vi "Extrae_Wait.vi"(10 "String":string="Wait for Temperature, Field, Timeout 300sec, Continue") -> (1 "Array":string[](array[string]))   [LabVIEW 2017]
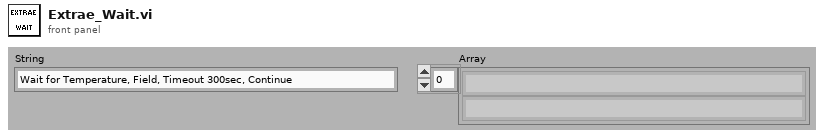
[diagram p1: front panel]
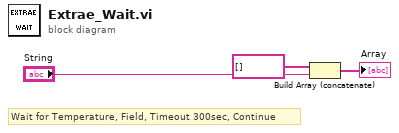
[diagram p0: block diagram]
diagram:
  # "Wait for Temperature, Field, Timeout 300sec, Continue"
  n1 = Build Array (concatenate)(string[] [] ("Array I"), "String") -> (→"Array":string[])
